vi "PidWIthLabVIewPid.vi"   [LabVIEW 2018]
uses:
  <vilib>/addons/control/pid/pid.llb/PID (DBL).vi
  <vilib>/addons/control/pid/NI_PID_pid.lvlib
  <vilib>/addons/control/pid/NI_PID_autopid.lvlib
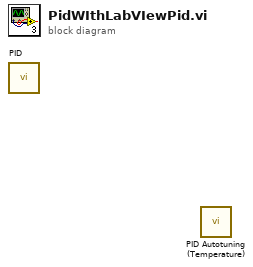
[diagram p0: block diagram]
diagram:
  n1 = call-poly <vilib>:"PID.vi"() -> ()  [unwired: 10 in, 2 out]
  n2 = call <vilib>:"PID Autotuning (Temperature).vi"() -> ()  [unwired: 16 in, 4 out]
